vi "字符串 时间 转换.vi"() -> ()   [LabVIEW 2023]
panel:
  out "毫秒":dbl
  out "秒":i32
  out "分钟":i32
  out "小时":i32
  out "日":i32
  out "月":i32
  out "年":i32
  out "output 1":timestamp
  out "String":string
  out "concatenated string":string
  out "current time 2":timestamp
  out "date/time string":string
  out "current time":timestamp
  out "time string":string
  out "date string":string
  # "字符串 时间 转换"
  # "提取时间 量"
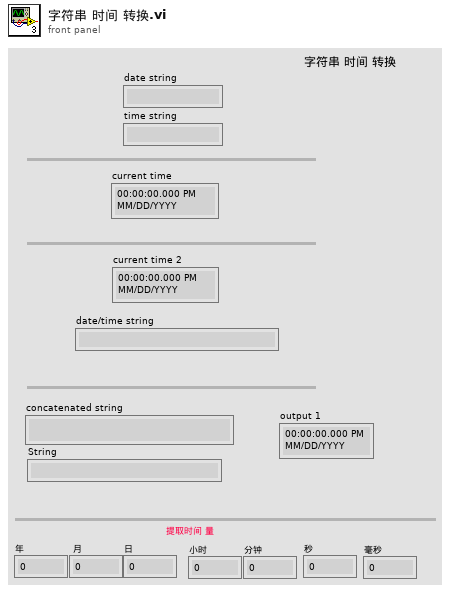
[diagram p1: front panel]
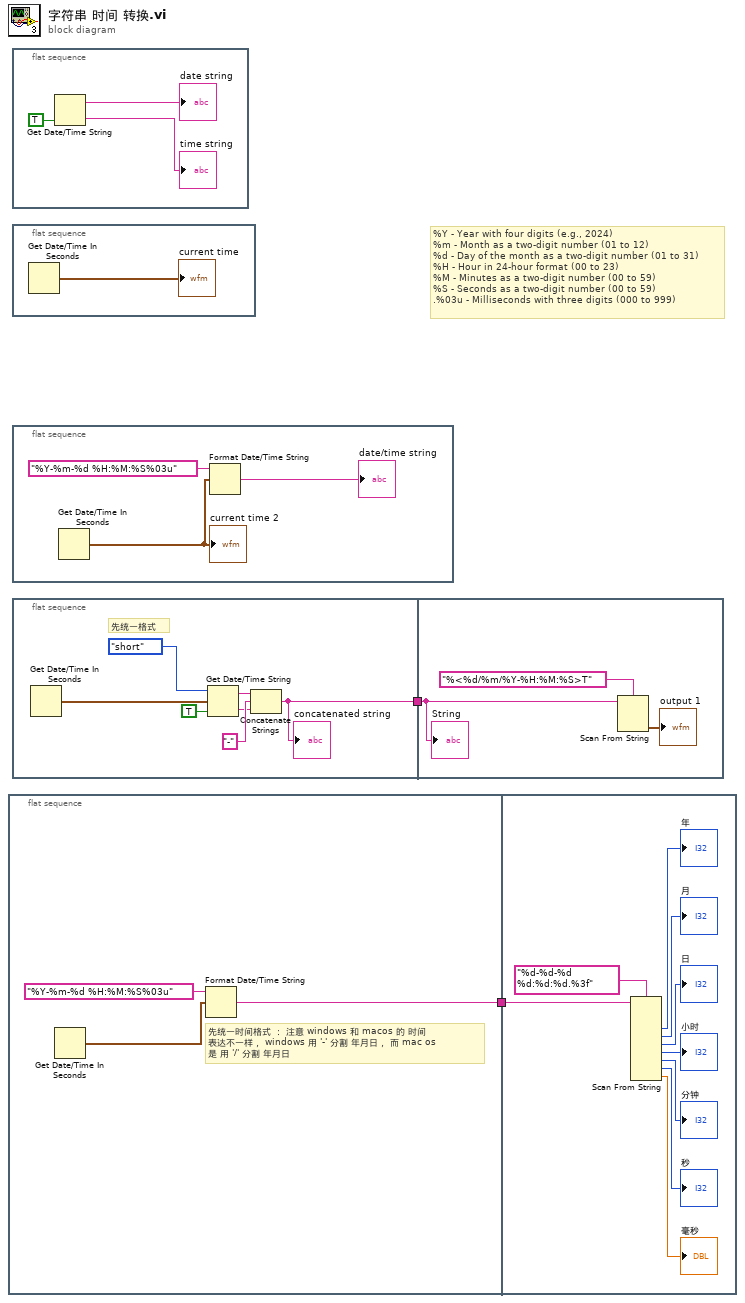
[diagram p0: block diagram]
diagram:
  # "%Y - Year with four digits (e.g., 2024)\n%m - Month as a two-digit number (01 to 12)\n%d - Day of the month as a two-digit number (01 to 31)\n%H - Hour in 24-hour format (00 to 23)\n%M - Minutes as a two-digit number (00 to 59)\n%S - Seconds as a two-digit number (00 to 59)\n.%03u - Milliseconds with three digits (000 to 999)"
  n1 = flat-sequence {
    tunnel: [w3] -> w1
    tunnel: w1 -> [w14]
    frame #0 {
      # "先统一时间格式 ： 注意 windows 和 macos 的 时间\n表达不一样， windows 用 '-' 分割 年月日， 而 mac os\n是 用 '/' 分割 年月日"
      n2 = Get Date/Time In Seconds() -> (seconds since 1Jan1904=w4:timestamp)
      n3 = Format Date/Time String(time format string (%c)="%Y-%m-%d %H:%M:%S%03u", seconds (now)=w4) -> (date/time string=w3:string)  [unwired: 1 in]
    }
    frame #1 {
      n4 = Scan From String(format string="%d-%d-%d %d:%d:%d.%3f", input string=w14) -> (output 1=→"年":i32, output 2=→"月":i32, output 3=→"日":i32, output 4=→"小时":i32, output 5=→"分钟":i32, output 6=→"秒":i32, output 7=→"毫秒":dbl)  [unwired: 9 in, 3 out]
    }
  }
  n5 = flat-sequence {
    frame #0 {
      n6 = Get Date/Time String(want seconds? (F)=TRUE) -> (date string=→"date string":string, time string=→"time string":string)  [unwired: 2 in]
    }
  }
  n7 = flat-sequence {
    frame #0 {
      n8 = Get Date/Time In Seconds() -> (seconds since 1Jan1904=→"current time":timestamp)
    }
  }
  n9 = flat-sequence {
    frame #0 {
      n10 = Get Date/Time In Seconds() -> (seconds since 1Jan1904=w19:timestamp)
      "current time 2" <- w19
      n11 = Format Date/Time String(time format string (%c)="%Y-%m-%d %H:%M:%S%03u", seconds (now)=w19) -> (date/time string=→"date/time string":string)  [unwired: 1 in]
    }
  }
  n12 = flat-sequence {
    tunnel: [w22] -> w2
    tunnel: w2 -> [w30]
    frame #0 {
      # "先统一格式"
      n13 = Get Date/Time In Seconds() -> (seconds since 1Jan1904=w27:timestamp)
      n14 = Get Date/Time String(date format (0)=enum16{"short", "long", "abbreviated"}."short", seconds (now)=w27, want seconds? (F)=TRUE) -> (date string=w25:string, time string=w23:string)
      n15 = Concatenate Strings(w25, "-", w23) -> (w22:string)
      "concatenated string" <- w22
    }
    frame #1 {
      n16 = Scan From String(format string="%<%d/%m/%Y-%H:%M:%S>T", input string=w30) -> (output 1=→"output 1":timestamp)  [unwired: 3 in, 3 out]
      "String" <- w30
    }
  }
